vi "Image Processing1.vi"() -> ()   [LabVIEW 2016]
uses:
  <vilib>/visionFPGA/Controls/IMAQ FPGA Image Size.ctl
  <vilib>/rvi/Emulation/niFpgaSctlEmulationGetInTimedLoop.vi
  <vilib>/rvi/Emulation/niFpgaProcessEmulError.vi
  <vilib>/rvi/Emulation/niFpgaGetClockAttributes.vi
  <vilib>/rvi/Emulation/niFpgaEmulationReportErrorSimple.vi
  <vilib>/rvi/eio/common/nirviEmuTemplateMethod_errors.vi
  <vilib>/rvi/interface/RandomDataEmulation/niFpgaRandomDataHandleErrors.vi
  <vilib>/rvi/DataTransferAndStorage/Container/Common/niFpgaContainerGetUniqueNameForEmu.vi
  <vilib>/rvi/DataTransferAndStorage/Container/Common/niFpgaContainerSetEmuInfo.vi
  <vilib>/rvi/eio/common/nirviEmuReportErrorAndStop.vi
  <vilib>/rvi/DataTransferAndStorage/Container/Common/niFpgaContainerExecOnDevCompGetState.vi
  <vilib>/rvi/Emulation/niFpgaEmulationIsFPGAContextNoSignature.vi
  <vilib>/rvi/errors/niFpgaSetErrorForExecOnDevCompSimple.vi
  <vilib>/rvi/FIFO/Fifo_Resource/nirvififoEmulationSetSize.vi
  <vilib>/rvi/FIFO/Fifo_Resource/nirviFifoEmulationQueueMgr.vi
  <instcachedir>/0/nirviFifoEmulationQueueMgr_E5CAEC123FF24DC58D834DCA3CDAA9B5.lvgen/nirviFifoEmulationQueueMgr_E5CAEC123FF24DC58D834DCA3CDAA9B5_002.vi
  <vilib>/rvi/FIFO/Fifo_Resource/nirvififoEmulationDetermineInputValidOut.vi
  <vilib>/rvi/FIFO/Fifo_Resource/nirvififoEmulationCreateLock.vi
  <vilib>/rvi/FIFO/Fifo_Resource/nirvififoEmulationObtainLock.vi
  <vilib>/rvi/FIFO/Fifo_Resource/nirvififoEmulationReleaseLock.vi
  <vilib>/rvi/occurrence/nirviWaitOnOccurrenceBase.vi
  <vilib>/rvi/errors/nirviReportUnexpectedCaseInternalError.vi
  <vilib>/rvi/errors/nirviReportUnexpectedCaseInternalError (U32).vi
  <vilib>/Utility/error.llb/Clear Errors.vi
  <vilib>/rvi/Emulation/niFpgaCriticalErrorInLSC.vi
  <vilib>/eio/EIONode/EIONode.xnode
  <vilib>/rvi/DataTransferAndStorage/Container/XNode/niFpgaContainer.xnode
  <vilib>/rvi/interface/RandomDataEmulation/nirviRandomDataFpgaReadWriteTemplate.vi
  <vilib>/rvi/LocalResourceManager/LocalResourceManager.xnode
  <vilib>/rvi/FIFO/Fifo_Resource/niFpgaFifoEmulationRefIn.vi
panel:
  out "col 3":u16
  out "row 3":u16
  out "col 2":u16
  out "row 2":u16
  out "row":u16
  out "col":u16
  out "OutCount":u32
  out "InCount":u32
  out "deHeight":u16=240
  out "deWidth":u16=320
  out "Count":u32
  out "OutputType":u8
  out "CanSendImage":bool=TRUE
  out "Mode LED Status":bool=TRUE
  out "Radio LED Status":bool=TRUE
  out "outputExtreme2":bool=TRUE
  out "outputExtreme1":bool=TRUE
  out "outputDOG2":bool=TRUE
  out "outputDOG1":bool=TRUE
  out "Ready For Output":bool=TRUE
  out "StartOfImage":bool=TRUE
  in  "Image Size":T1={"Width"=640, "Height"=480}
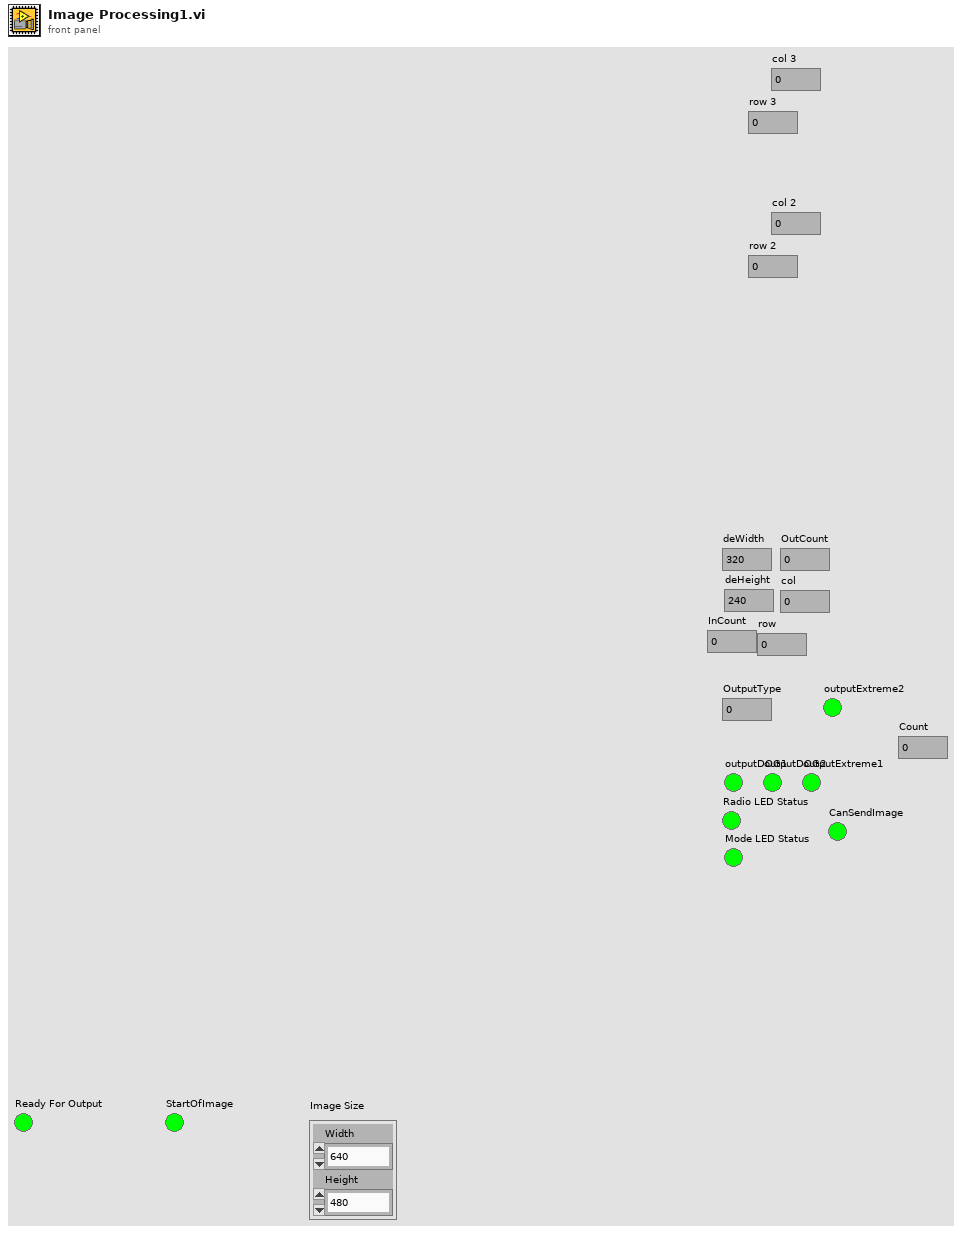
[diagram p1: front panel]
types:
  T1 = typedef "IMAQ FPGA Image Size.ctl" = cluster{"Width":u32, "Height":u32}
  T2 = cluster{"curCol":u16, "curRow":u16, "Width":u32, "Height":u32, "Data Out":fxp<+,8,8>, bool}
  T3 = cluster{"curCol":u16, "curRow":u16, "Width":u32, "Height":u32, "GaussianFilterData out":fxp<+,12,12>, "DV out":bool}
  T4 = cluster{"t":u32, "t":u32, "deWidth":u16, "deHeight":u16, "GaussianFilterData out":fxp<+,12,12>, "DV out":bool}
  T5 = cluster{"t":u32, "t":u32, "deWidth":u16, "deHeight":u16, "Data Out":fxp<+,8,8>, "DV out":bool}
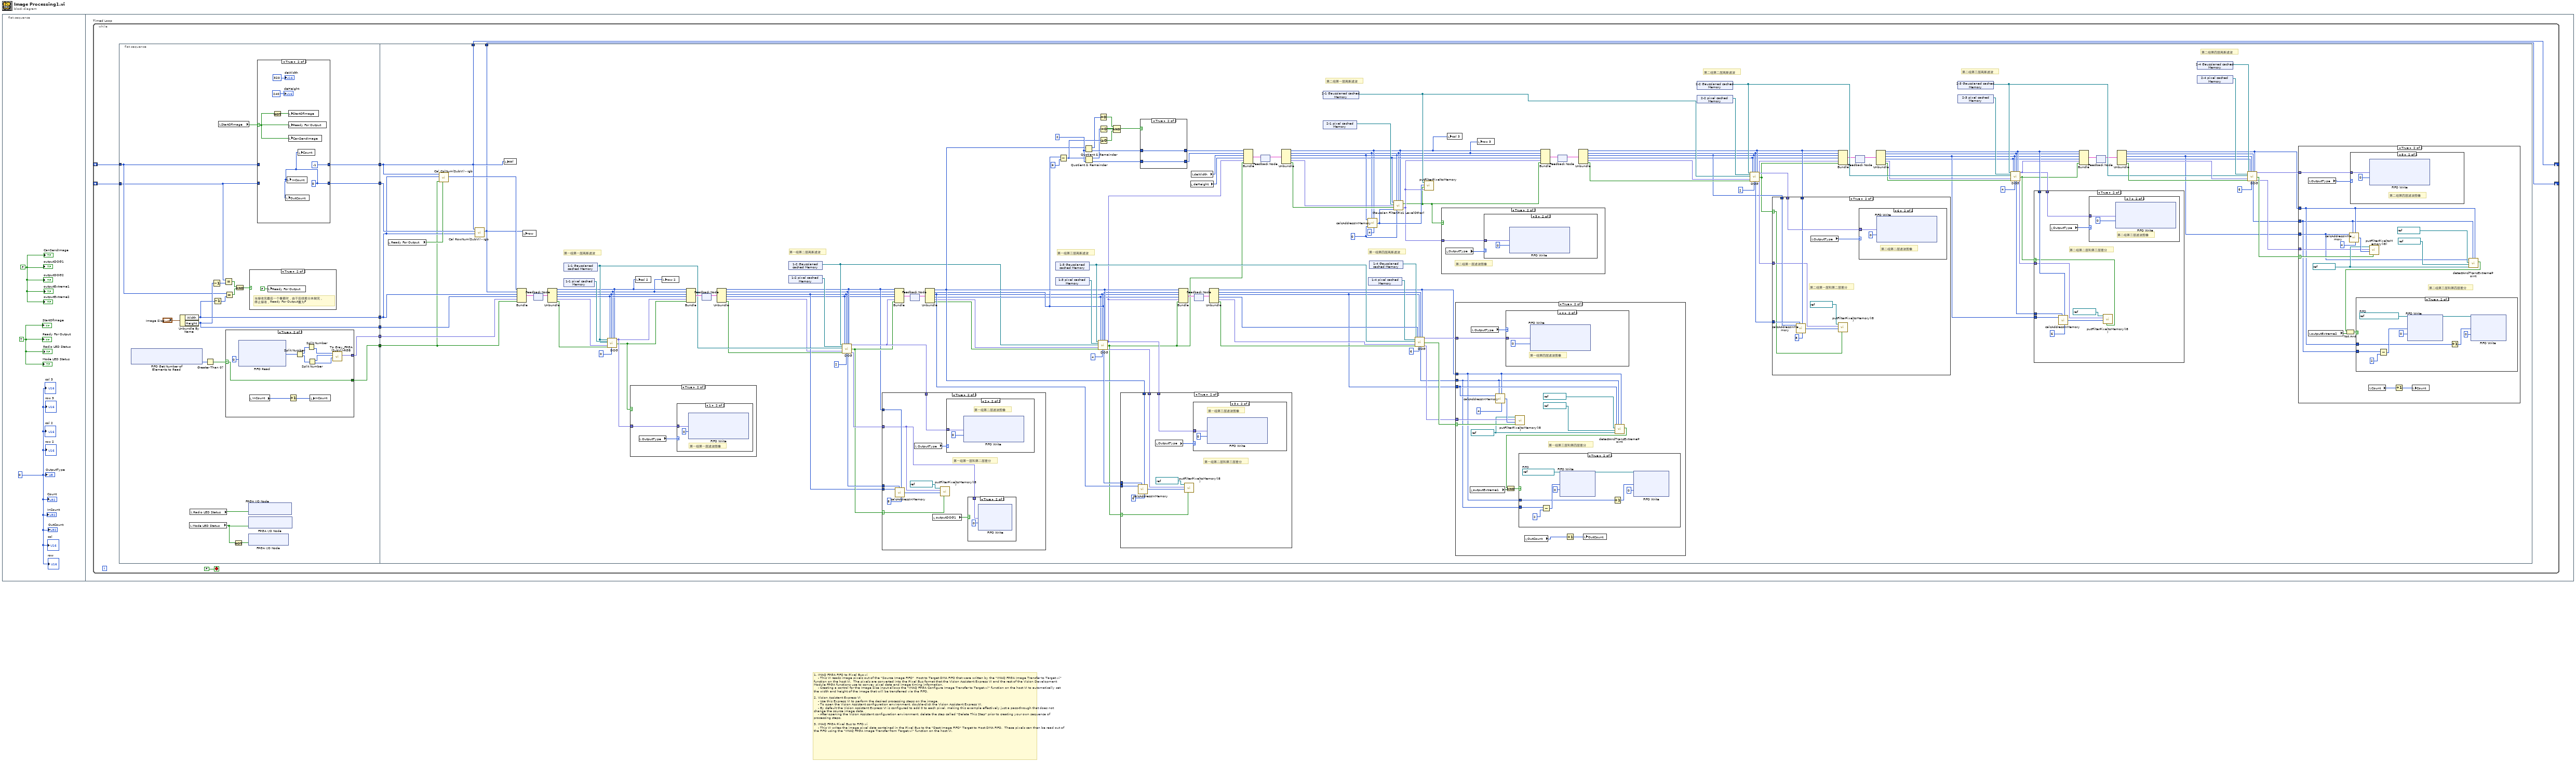
[diagram p0: block diagram]
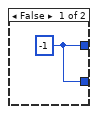
[diagram p10: hidden frame]
diagram:
  # "1. IMAQ FPGA FIFO to Pixel Bus.vi\n    - This VI reads image pixels out of the \"Source Image FIFO\"  Host to Target DMA FIFO that were written by the \"IMAQ FPGA Image Transfer to Target.vi\" function on the host VI.  The pixels are converted into the Pixel Bus format that the Vision Assistant Express VI and the rest of the Vision Development Module FPGA functions use to convey pixel data and image timing information.\n    - Creating a control for the Image Size input allows the \"IMAQ FPGA Configure Image Transfer to Target.vi\" function on the host VI to automatically set the width and height of the image that will be transferred via the FIFO.\n\n2. Vision Assistant Express VI\n    - Use this Express VI to perform the desired processing steps on the image.\n    - To open the Vision Assistant configuration environment, double-click the Vision Assistant Express VI.\n    - By default the Vision Assistant Express VI is configured to add 0 to each pixel, making this example effectively just a pass-through that does not change the source image data.\n    - After opening the Vision Assistant configuration environment, delete the step called \"Delete This Step\" prior to creating your own sequence of processing steps.\n\n3. IMAQ FPGA Pixel Bus to FIFO.vi\n    - This VI writes the image pixel data contained in the Pixel Bus to the \"Dest Image FIFO\" Target to Host DMA FIFO.  These pixels can then be read out of the FIFO using the \"IMAQ FPGA Image Transfer from Target.vi\" function on the host VI."
  n1 = flat-sequence {
    frame #0 {
      w2 = FALSE
      w1 = i16 0
      w3 = TRUE ("Ready For Output")
      "StartOfImage" <- w3
      "Ready For Output" <- w3
      "outputDOG1" <- w2
      "outputDOG2" <- w2
      "outputExtreme1" <- w2
      "outputExtreme2" <- w2
      "Radio LED Status" <- w3
      "Mode LED Status" <- w3
      "CanSendImage" <- w2
      "OutputType" <- w1
      "Count" <- w1
      "InCount" <- w1
      "OutCount" <- w1
      "col" <- w1
      "row" <- w1
      "col 2" <- w1
      "row 2" <- w1
      "col 3" <- w1
      "row 3" <- w1
    }
    frame #1 {
      n2 = while "Timed Loop" {
        shift-right: [w4] -> _
        shift-left: _ -> [w8]
        shift-right: [w5] -> _
        shift-left: _ -> [w9]
        stop <- FALSE stop-if-true
        n3 = flat-sequence {
          tunnel: [w29] -> w14
          tunnel: [w27] -> w13
          tunnel: [w26] -> w12
          tunnel: [w28] -> w11
          tunnel: [w22] -> w7
          tunnel: [w21] -> w6
          tunnel: w8 -> [w23]
          tunnel: w9 -> [w24]
          tunnel: [w61] -> w5
          tunnel: [w60] -> w4
          tunnel: w6 -> [w116]
          tunnel: w7 -> [w61]
          tunnel: w11 -> [w110]
          tunnel: w12 -> [w112]
          tunnel: w13 -> [w113]
          tunnel: w14 -> [w111]
          frame #0 {
            n4 = xnode ("FIFO Get Number of Elements to Read")() -> ("Number of Elements to Read"=w16:u32)  [unwired: 1 in, 1 out]
            n5 = Unbundle By Name("Image Size") -> ("Width"=w27:u32, "Height"=w26:u32)
            n6 = local read "Mode LED Status"() -> (w19:bool)
            n7 = local read "Radio LED Status"() -> (w17:bool)
            n8 = Greater Than 0?(x=w16) -> (x > 0?=w15:bool)
            n9 = Decrement(x=w26) -> (x-1=w32:u32)
            n10 = Decrement(x=w27) -> (x-1=w31:u32)
            n11 = local read "StartOfImage"() -> (w25:bool)
            n12 = Equal?(x=w23, y=w32) -> (x = y?=w34:bool)
            n13 = Equal?(x=w24, y=w31) -> (x = y?=w33:bool)
            n14 = case shown="True" w15 {
              selector: w15 -> [w35 w38]
              tunnel: [_ w39] -> w29
              tunnel: [w35 w38] -> w28
              frame False {
              }
              frame True {
                n15 = xnode ("FIFO Read")("Timeout"=0) -> ("Element"=w46:u32)  [unwired: 1 in, 2 out]
                n16 = local read "InCount"() -> (w36:u32)
                n17 = Increment(x=w36) -> (x+1=w37:u32)
                n18 = Split Number(x=w46) -> (hi(x)=w44:u16, lo(x)=w45:u16)
                n19 = Split Number(x=w44) -> (lo(x)=w43:u8)  [unwired: 1 out]
                n20 = Split Number(x=w45) -> (hi(x)=w42:u8, lo(x)=w41:u8)
                n21 = local write "InCount"(w37) -> ()
                n22 = call "To Gray_FPGA (SubVI)-RGB.vi"("B"=w41, "G"=w42, "R"=w43) -> ("Data Out"=w39:fxp<+,8,8>)  [unwired: 8 in]
              }
            }
            n23 = Not(x=w19) -> (.not. x?=w18:bool)
            n24 = And(x=w34, y=w33) -> (x .and. y?=w30:bool)
            n25 = xnode "FPGA I/O Node"("Radio LED Green"=w17) -> ()  [unwired: 1 in, 1 out]
            n26 = xnode "FPGA I/O Node"("Mode LED Green"=w19) -> ()  [unwired: 1 in, 1 out]
            n27 = xnode "FPGA I/O Node"("Mode LED Red"=w18) -> ()  [unwired: 1 in, 1 out]
            n28 = case shown="True" w30 {
              frame False {
              }
              frame True {
                # "当接收完最后一个像素时，由于后续差分未做完，\n停止接收，Ready For Output置为F"
                n29 = local write "Ready For Output"(FALSE ("Ready For Output")) -> ()
              }
            }
            n30 = case shown="True" w25 {
              selector: w25 -> [_ w52]
              tunnel: w24 -> [w48 _]
              tunnel: w23 -> [w47 _]
              tunnel: [w48 i16 -1] -> w22
              tunnel: [w47 w49] -> w21
              frame False {
              }
              frame True {
                w49 = i16 0
                n31 = Not(x=w52) -> (.not. x?=w53:bool)
                n32 = local write "OutCount"(w49) -> ()
                n33 = local write "InCount"(w49) -> ()
                n34 = local write "StartOfImage"(w53) -> ()
                n35 = local write "Ready For Output"(w52) -> ()
                n36 = local write "CanSendImage"(w52) -> ()
                n37 = local write "Count"(w49) -> ()
                "deWidth" <- i16 320
                "deHeight" <- i16 240
              }
            }
          }
          frame #1 {
            w146 = u32 2 ("y")
            w151 = u8 0 ("delayRowCount")
            # "第一组第一层高斯滤波"
            # "第一组第二层高斯滤波"
            # "第一组第三层高斯滤波"
            # "第二组第一层高斯滤波"
            # "第一组第四层高斯滤波"
            # "第二组第二层高斯滤波"
            # "第二组第三层高斯滤波"
            # "第二组第四层高斯滤波"
            n38 = local read "Ready For Output"() -> (w115:bool)
            n39 = call "Cal ColNum(SubVI) - rgb.vi"("Ready For Input"=w115, "DV"=w110, "Width"=w113, "preCol"=w61) -> ("curCol"=w114:u16)  [unwired: 7 in]
            n40 = call "Cal RowNum(SubVI) - rgb.vi"("Width"=w113, "preRow"=w116, "preCol"=w61) -> ("curRow"=w60:u16)  [unwired: 8 in]
            n41 = local write "col"(w61) -> ()
            n42 = Bundle("curCol"=w114, "curRow"=w60, "Width"=w113, "Height"=w112, "Data Out"=w111, w110) -> (w109:T2)  [unwired: 1 in]
            n43 = local write "row"(w60) -> ()
            n44 = feedback #1() -> (w108:T2)  [unwired: 1 in]
            n45 = feedback-in #1(w109) -> ()
            n46 = Unbundle(w108) -> ("curCol"=w59:u16, "curRow"=w58:u16, "Width"=w120:u32, "Height"=w119:u32, "Data Out"=w126:fxp<+,8,8>, w123:bool)
            n47 = xnode "1-1 Gaussianed cached Memory"() -> ("Memory Out"=w98:refnum<k21>)
            n48 = xnode "1-1 pixel cached Memory"() -> ("Memory Out"=w125:refnum<k21>)
            n49 = call "DOG.vi"("Gaussianed cached Memory"=w98, "pixel cached Memory"=w125, "preGaussianed cached Memory"=w98, "Data in"=w126, "DV in"=w123, "Height"=w119, "Width"=w120, "DelayRowCount"=i16 0, "Rows"=w58, "Cols"=w59) -> ("GaussianFilterData out"=w118:fxp<+,12,12>, "DV out"=w117:bool)  [unwired: 6 in, 2 out]
            n50 = case shown="True" w117 {
              tunnel: w118 -> [_ w199]
              frame False {
              }
              frame True {
                n51 = local read "OutputType"() -> (w198:u8)
                n52 = case shown="1" w198 {
                  tunnel: w199 -> [_ w200]
                  frame 0, Default {
                  }
                  frame 1 {
                    # "第一组第一层滤波图像"
                    n53 = xnode ("FIFO Write")("Element"=w200, "Timeout"=0) -> ()  [unwired: 1 in, 2 out]
                  }
                }
              }
            }
            n54 = local write "col 2"(w59) -> ()
            n55 = local write "row 2"(w58) -> ()
            n56 = Bundle("curCol"=w59, "curRow"=w58, "Width"=w120, "Height"=w119, "GaussianFilterData out"=w118, "DV out"=w117) -> (w122:T3)  [unwired: 1 in]
            n57 = feedback #2() -> (w121:T3)  [unwired: 1 in]
            n58 = feedback-in #2(w122) -> ()
            n59 = Unbundle(w121) -> ("curCol"=w97:u16, "curRow"=w96:u16, "Width"=w95:u32, "Height"=w94:u32, "GaussianFilterData out"=w93:fxp<+,12,12>, "DV out"=w92:bool)
            n60 = xnode "1-2 Gaussianed cached Memory"() -> ("Memory Out"=w99:refnum<k21>)
            n61 = xnode "1-2 pixel cached Memory"() -> ("Memory Out"=w133:refnum<k21>)
            n62 = call "DOG.vi"("Gaussianed cached Memory"=w99, "pixel cached Memory"=w133, "preGaussianed cached Memory"=w98, "Data in"=w93, "DV in"=w92, "Height"=w94, "Width"=w95, "DelayRowCount"=i16 2, "Rows"=w96, "Cols"=w97) -> ("out Row"=w131:u16, "GaussianFilterData out"=w128:fxp<+,12,12>, "DV out"=w127:bool, "DOG Out"=w132:fxp<+/-,13,13>)  [unwired: 6 in]
            n63 = case shown="True" w127 {
              selector: w127 -> [_ w205]
              tunnel: w128 -> [_ w212]
              tunnel: w132 -> [_ w203]
              tunnel: w95 -> [_ w211]
              tunnel: w131 -> [_ w210]
              tunnel: w97 -> [_ w209]
              frame False {
              }
              frame True {
                # "第一组第一层和第二层差分"
                n64 = call "calcAddressInMemory.vi"("Width"=w211, "Rows"=w210, "Cols"=w209, "divider"=u8 8) -> ("addressInMemory"=w207:u16)  [unwired: 5 in]
                n65 = local read "OutputType"() -> (w204:u8)
                n66 = local read "outputDOG1"() -> (w202:bool)
                n67 = call "putFilterPixeltoMemory(I8).vi"("DV in"=w205, "addressInMemory"=w207, "Data In"=w203, "Memory in"=refnum<k21> "DOG1-1") -> ()  [unwired: 8 in]
                n68 = case shown="2" w204 {
                  tunnel: w212 -> [_ w215]
                  frame 0, Default {
                  }
                  frame 2 {
                    # "第一组第二层滤波图像"
                    n69 = xnode ("FIFO Write")("Element"=w215, "Timeout"=0) -> ()  [unwired: 1 in, 2 out]
                  }
                }
                n70 = case shown="True" w202 {
                  tunnel: w203 -> [_ w214]
                  frame False {
                  }
                  frame True {
                    n71 = xnode ("FIFO Write")("Element"=w214, "Timeout"=0) -> ()  [unwired: 1 in, 2 out]
                  }
                }
              }
            }
            n72 = Bundle("curCol"=w97, "curRow"=w96, "Width"=w95, "Height"=w94, "GaussianFilterData out"=w128, "DV out"=w127) -> (w130:T3)  [unwired: 1 in]
            n73 = feedback #3() -> (w129:T3)  [unwired: 1 in]
            n74 = feedback-in #3(w130) -> ()
            n75 = Unbundle(w129) -> ("curCol"=w105:u16, "curRow"=w104:u16, "Width"=w103:u32, "Height"=w102:u32, "GaussianFilterData out"=w101:fxp<+,12,12>, "DV out"=w100:bool)
            n76 = xnode "1-3 pixel cached Memory"() -> ("Memory Out"=w149:refnum<k21>)
            n77 = xnode "1-3 Gaussianed cached Memory"() -> ("Memory Out"=w163:refnum<k21>)
            n78 = Subtract(x=w104, y=i16 6) -> (x-y=w139:u16)
            n79 = Quotient & Remainder(x=w105, y=w146) -> (x-y*floor(x/y)=w138:u32, floor(x/y)=w140:u32)
            n80 = Quotient & Remainder(x=w139, y=w146) -> (x-y*floor(x/y)=w137:u32, floor(x/y)=w141:u32)
            n81 = call "DOG.vi"("Gaussianed cached Memory"=w163, "pixel cached Memory"=w149, "preGaussianed cached Memory"=w99, "Data in"=w101, "DV in"=w100, "Height"=w102, "Width"=w103, "DelayRowCount"=i16 4, "Rows"=w104, "Cols"=w105) -> ("out Row"=w135:u16, "GaussianFilterData out"=w87:fxp<+,12,12>, "DV out"=w86:bool, "DOG Out"=w136:fxp<+/-,13,13>)  [unwired: 6 in]
            n82 = Equal To 0?(x=w138) -> (x = 0?=w145:bool)
            n83 = Equal To 0?(x=w137) -> (x = 0?=w144:bool)
            n84 = Greater Or Equal To 0?(x=w139) -> (x >= 0?=w143:bool)
            n85 = Compound Arithmetic op=AND(w145, w144, w143) -> (w142:bool)
            n86 = case shown="True" w86 {
              selector: w86 -> [_ w221]
              tunnel: w87 -> [_ w229]
              tunnel: w136 -> [_ w222]
              tunnel: w135 -> [_ w225]
              tunnel: w103 -> [_ w224]
              tunnel: w105 -> [_ w223]
              frame False {
              }
              frame True {
                # "第一组第二层和第三层差分"
                n87 = call "calcAddressInMemory.vi"("Width"=w224, "Rows"=w225, "Cols"=w223, "divider"=u8 6) -> ("addressInMemory"=w227:u16)  [unwired: 5 in]
                n88 = local read "OutputType"() -> (w220:u8)
                n89 = call "putFilterPixeltoMemory(I8).vi"("DV in"=w221, "addressInMemory"=w227, "Data In"=w222, "Memory in"=refnum<k21> "DOG1-2") -> ()  [unwired: 8 in]
                n90 = case shown="3" w220 {
                  tunnel: w229 -> [_ w230]
                  frame 0, Default {
                  }
                  frame 3 {
                    # "第一组第三层滤波图像"
                    n91 = xnode ("FIFO Write")("Element"=w230, "Timeout"=0) -> ()  [unwired: 1 in, 2 out]
                  }
                }
              }
            }
            n92 = case shown="True" w142 {
              tunnel: [w217 w219] -> w91
              tunnel: w140 -> [_ w219]
              tunnel: [w217 w218] -> w90
              tunnel: w141 -> [_ w218]
              frame False {
                w217 = i16 -1 ("t")
              }
              frame True {
              }
            }
            n93 = Bundle("curCol"=w105, "curRow"=w104, "Width"=w103, "Height"=w102, "GaussianFilterData out"=w87, "DV out"=w86) -> (w107:T3)  [unwired: 1 in]
            n94 = local read "deHeight"() -> (w89:u16)
            n95 = local read "deWidth"() -> (w88:u16)
            n96 = feedback #4() -> (w106:T3)  [unwired: 1 in]
            n97 = feedback-in #4(w107) -> ()
            n98 = Unbundle(w106) -> ("curCol"=w153:u16, "curRow"=w167:u16, "Width"=w155:u32, "Height"=w166:u32, "GaussianFilterData out"=w169:fxp<+,12,12>, "DV out"=w168:bool)
            n99 = Bundle("t"=w91, "t"=w90, "deWidth"=w88, "deHeight"=w89, "GaussianFilterData out"=w87, "DV out"=w86) -> (w85:T4)  [unwired: 1 in]
            n100 = feedback #5() -> (w84:T4)  [unwired: 1 in]
            n101 = feedback-in #5(w85) -> ()
            n102 = Unbundle(w84) -> ("t"=w57:u32, "t"=w56:u32, "deWidth"=w81:u16, "deHeight"=w80:u16, "GaussianFilterData out"=w159:fxp<+,12,12>, "DV out"=w160:bool)
            n103 = xnode "2-1 Gaussianed cached Memory"() -> ("Memory Out"=w174:refnum<k21>)
            n104 = xnode "2-1 pixel cached Memory"() -> ("Memory Out"=w158:refnum<k21>)
            n105 = call "calcAddressInMemory.vi"("Width"=w81, "Rows"=w56, "delayRowCount"=w151, "Cols"=w57, "divider"=u8 4) -> ("addressInMemory"=w152:u16)  [unwired: 4 in]
            n106 = xnode "1-4 pixel cached Memory"() -> ("Memory Out"=w164:refnum<k21>)
            n107 = xnode "1-4 Gaussianed cached Memory"() -> ("Memory Out"=w165:refnum<k21>)
            n108 = call "Gaussian Filter(Pic1 LevelOther).vi"("Height"=w80, "Width"=w81, "Rows"=w56, "Cols"=w57, "Memory in"=w158, "Data in"=w159, "DV in"=w160, "Address In"=w152, "DelayRowCount"=w151) -> ("DV out"=w78:bool, "Data Out"=w79:fxp<+,8,8>)  [unwired: 4 in, 1 out]
            n109 = call "DOG.vi"("Gaussianed cached Memory"=w165, "pixel cached Memory"=w164, "preGaussianed cached Memory"=w163, "Data in"=w169, "DV in"=w168, "Height"=w166, "Width"=w155, "DelayRowCount"=i16 6, "Rows"=w167, "Cols"=w153) -> ("out Row"=w154:u16, "GaussianFilterData out"=w161:fxp<+,12,12>, "DV out"=w157:bool, "DOG Out"=w156:fxp<+/-,13,13>)  [unwired: 6 in]
            n110 = call "putFilterPixeltoMemory.vi"("Data In"=w79, "DV in"=w78, "addressInMemory"=w152, "Memory in"=w174) -> ()
            n111 = case shown="True" w78 {
              tunnel: w79 -> [_ w233]
              frame False {
              }
              frame True {
                # "第二组第一层滤波图像"
                n112 = local read "OutputType"() -> (w232:u8)
                n113 = case shown="5" w232 {
                  tunnel: w233 -> [_ w234]
                  frame 0, Default {
                  }
                  frame 5 {
                    n114 = xnode ("FIFO Write")("Element"=w234, "Timeout"=0) -> ()  [unwired: 1 in, 2 out]
                  }
                }
              }
            }
            n115 = local write "col 3"(w57) -> ()
            n116 = case shown="True" w157 {
              selector: w157 -> [_ w248]
              tunnel: w161 -> [_ w252]
              tunnel: w156 -> [_ w249]
              tunnel: w155 -> [_ w247]
              tunnel: w154 -> [_ w241]
              tunnel: w153 -> [_ w242]
              frame False {
              }
              frame True {
                w244 = refnum<k21> "DOG1-3" ("Memory in")
                # "第一组第三层和第四层差分"
                n117 = local read "outputExtreme1"() -> (w239:bool)
                n118 = local read "OutputType"() -> (w243:u8)
                n119 = call "calcAddressInMemory.vi"("Width"=w247, "Rows"=w241, "Cols"=w242, "divider"=u8 4) -> ("addressInMemory"=w250:u16)  [unwired: 5 in]
                n120 = case shown="4" w243 {
                  tunnel: w252 -> [_ w263]
                  frame 0, Default {
                  }
                  frame 4 {
                    # "第一组第四层滤波图像"
                    n121 = xnode ("FIFO Write")("Element"=w263, "Timeout"=0) -> ()  [unwired: 1 in, 2 out]
                  }
                }
                n122 = call "putFilterPixeltoMemory(I8).vi"("DV in"=w248, "addressInMemory"=w250, "Data In"=w249, "Memory in"=w244) -> ()  [unwired: 8 in]
                n123 = local read "OutCount"() -> (w237:u32)
                n124 = Increment(x=w237) -> (x+1=w236:u32)
                n125 = local write "OutCount"(w236) -> ()
                n126 = call "detectAndTransExtremePoint.vi"("Col"=w242, "Row"=w241, "Level3 Memory"=w244, "Level2 Memory"=refnum<k21> "DOG1-2" ("Memory In"), "Level1 Memory"=refnum<k21> "DOG1-1" ("Memory In"), "Width"=w247) -> ("isExtreme?"=w238:bool)  [unwired: 5 in]
                n127 = And(x=w238, y=w239) -> (x .and. y?=w240:bool)
                n128 = case shown="True" w240 {
                  tunnel: w241 -> [_ w260]
                  tunnel: w242 -> [_ w254]
                  frame False {
                  }
                  frame True {
                    w253 = refnum<k21> "extreme FIFO"  # FIFO
                    n129 = Subtract(x=w260, y=u16 2) -> (x-y=w258:u16)
                    n130 = xnode ("FIFO Write")("Element"=w258, "Timeout"=0, "FIFO In"=w253) -> ("FIFO Out"=w256:refnum<k21>)  [unwired: 1 out]
                    n131 = Increment(x=w254) -> (x+1=w255:u16)
                    n132 = xnode ("FIFO Write")("Element"=w255, "Timeout"=0, "FIFO In"=w256) -> ()  [unwired: 2 out]
                  }
                }
              }
            }
            n133 = local write "row 3"(w56) -> ()
            n134 = Bundle("t"=w57, "t"=w56, "deWidth"=w81, "deHeight"=w80, "Data Out"=w79, "DV out"=w78) -> (w82:T5)  [unwired: 1 in]
            n135 = feedback #6() -> (w83:T5)  [unwired: 1 in]
            n136 = feedback-in #6(w82) -> ()
            n137 = Unbundle(w83) -> ("t"=w75:u32, "t"=w74:u32, "deWidth"=w73:u16, "deHeight"=w72:u16, "Data Out"=w173:fxp<+,8,8>, "DV out"=w172:bool)
            n138 = xnode "2-2 Gaussianed cached Memory"() -> ("Memory Out"=w181:refnum<k21>)
            n139 = xnode "2-2 pixel cached Memory"() -> ("Memory Out"=w175:refnum<k21>)
            n140 = call "DOG.vi"("Gaussianed cached Memory"=w181, "pixel cached Memory"=w175, "preGaussianed cached Memory"=w174, "Data in"=w173, "DV in"=w172, "Height"=w72, "Width"=w73, "DelayRowCount"=i16 2, "Rows"=w74, "Cols"=w75) -> ("out Row"=w170:u16, "GaussianFilterData out"=w71:fxp<+,12,12>, "DV out"=w70:bool, "DOG Out"=w171:fxp<+/-,13,13>)  [unwired: 6 in]
            n141 = case shown="True" w70 {
              selector: w70 -> [_ w265]
              tunnel: w171 -> [_ w266]
              tunnel: w71 -> [_ w273]
              tunnel: w75 -> [_ w269]
              tunnel: w170 -> [_ w268]
              tunnel: w73 -> [_ w267]
              frame False {
              }
              frame True {
                # "第二组第一层和第二层差分"
                n142 = call "calcAddressInMemory.vi"("Width"=w267, "Rows"=w268, "Cols"=w269, "divider"=u8 8) -> ("addressInMemory"=w271:u16)  [unwired: 5 in]
                n143 = local read "OutputType"() -> (w264:u8)
                n144 = call "putFilterPixeltoMemory(I8).vi"("DV in"=w265, "addressInMemory"=w271, "Data In"=w266, "Memory in"=refnum<k21> "DOG2-1") -> ()  [unwired: 8 in]
                n145 = case shown="6" w264 {
                  tunnel: w273 -> [_ w274]
                  frame 0, Default {
                  }
                  frame 6 {
                    # "第二组第二层滤波图像"
                    n146 = xnode ("FIFO Write")("Element"=w274, "Timeout"=0) -> ()  [unwired: 1 in, 2 out]
                  }
                }
              }
            }
            n147 = Bundle("t"=w75, "t"=w74, "deWidth"=w73, "deHeight"=w72, "GaussianFilterData out"=w71, "DV out"=w70) -> (w77:T4)  [unwired: 1 in]
            n148 = feedback #7() -> (w76:T4)  [unwired: 1 in]
            n149 = feedback-in #7(w77) -> ()
            n150 = Unbundle(w76) -> ("t"=w67:u32, "t"=w66:u32, "deWidth"=w65:u16, "deHeight"=w64:u16, "GaussianFilterData out"=w180:fxp<+,12,12>, "DV out"=w179:bool)
            n151 = xnode "2-3 Gaussianed cached Memory"() -> ("Memory Out"=w192:refnum<k21>)
            n152 = xnode "2-3 pixel cached Memory"() -> ("Memory Out"=w182:refnum<k21>)
            n153 = call "DOG.vi"("Gaussianed cached Memory"=w192, "pixel cached Memory"=w182, "preGaussianed cached Memory"=w181, "Data in"=w180, "DV in"=w179, "Height"=w64, "Width"=w65, "DelayRowCount"=i16 4, "Rows"=w66, "Cols"=w67) -> ("out Row"=w177:u16, "GaussianFilterData out"=w63:fxp<+,12,12>, "DV out"=w62:bool, "DOG Out"=w178:fxp<+/-,13,13>)  [unwired: 6 in]
            n154 = case shown="True" w62 {
              selector: w62 -> [_ w277]
              tunnel: w63 -> [_ w285]
              tunnel: w178 -> [_ w278]
              tunnel: w65 -> [_ w281]
              tunnel: w177 -> [_ w280]
              tunnel: w67 -> [_ w279]
              frame False {
              }
              frame True {
                # "第二组第二层和第三层差分"
                n155 = local read "OutputType"() -> (w276:u8)
                n156 = call "calcAddressInMemory.vi"("Width"=w281, "Rows"=w280, "Cols"=w279, "divider"=u8 6) -> ("addressInMemory"=w283:u16)  [unwired: 5 in]
                n157 = case shown="7" w276 {
                  tunnel: w285 -> [_ w287]
                  frame 0, Default {
                  }
                  frame 7 {
                    # "第二组第三层滤波图像"
                    n158 = xnode ("FIFO Write")("Element"=w287, "Timeout"=0) -> ()  [unwired: 1 in, 2 out]
                  }
                }
                n159 = call "putFilterPixeltoMemory(I8).vi"("DV in"=w277, "addressInMemory"=w283, "Data In"=w278, "Memory in"=refnum<k21> "DOG2-2") -> ()  [unwired: 8 in]
              }
            }
            n160 = Bundle("t"=w67, "t"=w66, "deWidth"=w65, "deHeight"=w64, "GaussianFilterData out"=w63, "DV out"=w62) -> (w68:T4)  [unwired: 1 in]
            n161 = feedback #8() -> (w69:T4)  [unwired: 1 in]
            n162 = feedback-in #8(w68) -> ()
            n163 = Unbundle(w69) -> ("t"=w185:u32, "t"=w184:u32, "deWidth"=w187:u16, "deHeight"=w191:u16, "GaussianFilterData out"=w194:fxp<+,12,12>, "DV out"=w193:bool)
            n164 = xnode "2-4 Gaussianed cached Memory"() -> ("Memory Out"=w195:refnum<k21>)
            n165 = xnode "2-4 pixel cached Memory"() -> ("Memory Out"=w196:refnum<k21>)
            n166 = call "DOG.vi"("Gaussianed cached Memory"=w195, "pixel cached Memory"=w196, "preGaussianed cached Memory"=w192, "Data in"=w194, "DV in"=w193, "Height"=w191, "Width"=w187, "DelayRowCount"=i16 6, "Rows"=w184, "Cols"=w185) -> ("out Row"=w186:u16, "GaussianFilterData out"=w189:fxp<+,12,12>, "DV out"=w190:bool, "DOG Out"=w188:fxp<+/-,13,13>)  [unwired: 6 in]
            n167 = case shown="True" w190 {
              selector: w190 -> [_ w298]
              tunnel: w189 -> [_ w304]
              tunnel: w188 -> [_ w297]
              tunnel: w187 -> [_ w296]
              tunnel: w186 -> [_ w294]
              tunnel: w185 -> [_ w295]
              frame False {
              }
              frame True {
                w299 = refnum<k21> "DOG2-3" ("Memory in")
                # "第二组第三层和第四层差分"
                n168 = local read "OutputType"() -> (w290:u8)
                n169 = local read "outputExtreme2"() -> (w291:bool)
                n170 = call "calcAddressInMemory.vi"("Width"=w296, "Rows"=w294, "Cols"=w295, "divider"=u8 4) -> ("addressInMemory"=w302:u16)  [unwired: 5 in]
                n171 = case shown="8" w290 {
                  tunnel: w304 -> [_ w306]
                  frame 0, Default {
                  }
                  frame 8 {
                    # "第二组第四层滤波图像"
                    n172 = xnode ("FIFO Write")("Element"=w306, "Timeout"=0) -> ()  [unwired: 1 in, 2 out]
                  }
                }
                n173 = local read "Count"() -> (w289:u32)
                n174 = call "putFilterPixeltoMemory(I8).vi"("DV in"=w298, "addressInMemory"=w302, "Data In"=w297, "Memory in"=w299) -> ()  [unwired: 8 in]
                n175 = Increment(x=w289) -> (x+1=w288:u32)
                n176 = local write "Count"(w288) -> ()
                n177 = call "detectAndTransExtremePoint.vi"("Col"=w295, "Row"=w294, "Level3 Memory"=w299, "Level2 Memory"=refnum<k21> "DOG2-2" ("Memory In"), "Level1 Memory"=refnum<k21> "DOG2-1" ("Memory In"), "Width"=w296) -> ("isExtreme?"=w292:bool)  [unwired: 5 in]
                n178 = Not And(1:w291, 2:w292) -> (0:w293:bool)
                n179 = case shown="True" w293 {
                  tunnel: w294 -> [_ w314]
                  tunnel: w295 -> [_ w308]
                  frame False {
                  }
                  frame True {
                    w307 = refnum<k21> "extreme FIFO dec"  # FIFO
                    n180 = Subtract(x=w314, y=u16 2) -> (x-y=w312:u16)
                    n181 = xnode ("FIFO Write")("Element"=w312, "Timeout"=0, "FIFO In"=w307) -> ("FIFO Out"=w310:refnum<k21>)  [unwired: 1 out]
                    n182 = Increment(x=w308) -> (x+1=w309:u32)
                    n183 = xnode ("FIFO Write")("Element"=w309, "Timeout"=0, "FIFO In"=w310) -> ()  [unwired: 2 out]
                  }
                }
              }
            }
          }
        }
      }
    }
  }
